vi "snr_test.vi"() -> ()   [LabVIEW 2017]
uses:
  <vilib>/measure/NI_MABase.lvlib
panel:
  in  "felharmonikus N":i32
  in  "noise (rms)":dbl format="%.2p"
  in  "zaj":bool
  out "kiolvasott frekvencia [Hz]":dbl
  in  "alh frekvencia [Hz]":dbl=10.0 format="%0.2p"
  in  "felh frekvencia [Hz]":dbl=10.0 format="%0.2p"
  out "Noise Integral":dbl
  out "Signal Integral":dbl
  out "SNR":dbl
  out "PSD":cluster{"f0":dbl, "df":dbl, "magnitude":dbl[]}[](graph)
  out "generált jel":waveform(dbl)(graph)
  in  "ablak szélesség [Hz]":dbl=20.0 format="%#_13g"
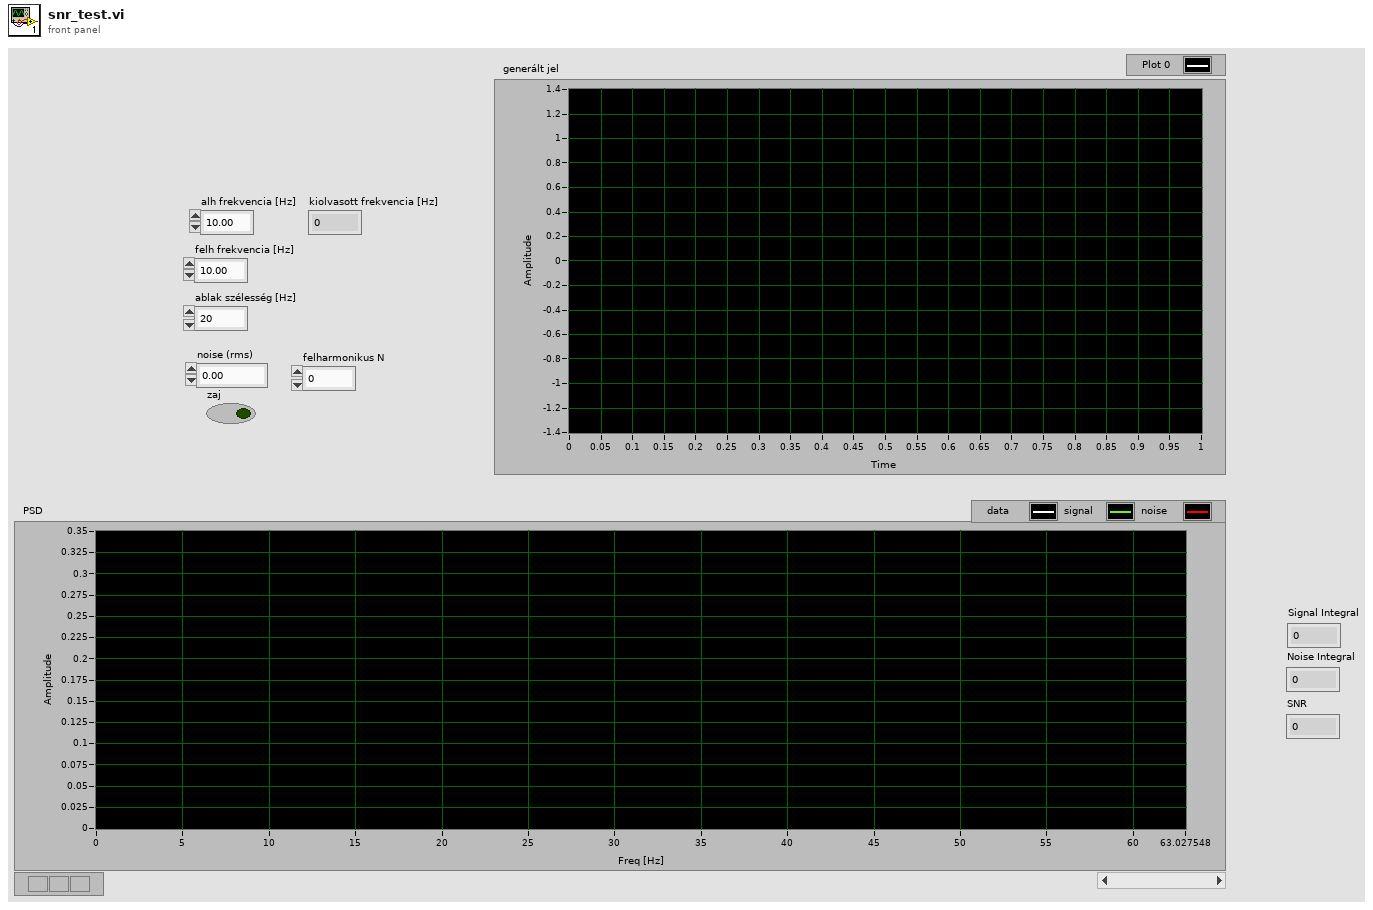
[diagram p1: front panel]
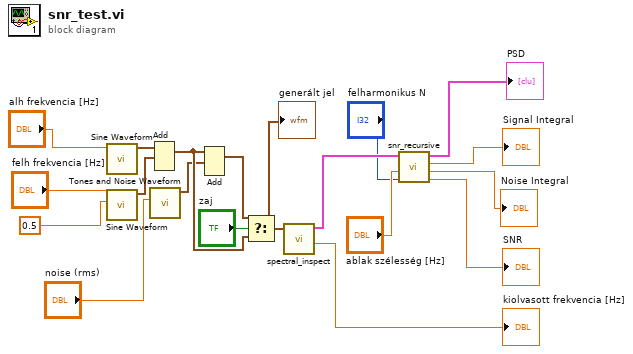
[diagram p0: block diagram]
diagram:
  n1 = call <vilib>:"Sine Waveform.vi"("frequency"="alh frekvencia [Hz]") -> ("signal out"=w17:waveform(dbl))  [unwired: 9 in, 1 out]
  n2 = call <vilib>:"Sine Waveform.vi"("amplitude"=0.5, "frequency"="felh frekvencia [Hz]") -> ("signal out"=w16:waveform(dbl))  [unwired: 8 in, 1 out]
  n3 = Add(1:w16, 2:w17) -> (0:w4:waveform(dbl))  [unwired: 1 in, 1 out]
  n4 = call <vilib>:"Tones and Noise Waveform.vi"("noise (rms)"="noise (rms)") -> ("signal out"=w3:waveform(dbl))  [unwired: 9 in, 1 out]
  n5 = Add(1:w3, 2:w4) -> (0:w5:waveform(dbl))  [unwired: 1 in, 1 out]
  n6 = Select(t=w5, s="zaj", f=w4) -> (s? t:f=w7:waveform(dbl))
  "generált jel" <- w7
  n7 = call "spectral_inspect.vi"("waveform"=w7) -> ("freq"=→"kiolvasott frekvencia [Hz]":dbl, "PSD"=w19:cluster{"f0":dbl, "df":dbl, "magnitude":dbl[]})  [unwired: 7 in, 2 out]
  n8 = call "snr_recursive.vi"("felharmonikus N"="felharmonikus N", "width [Hz]"="ablak szélesség [Hz]", "PSD"=w19) -> ("SNR"=→"SNR":dbl, "Noise Integral"=→"Noise Integral":dbl, "Signal Integral"=→"Signal Integral":dbl, "PSD"=→"PSD":cluster{"f0":dbl, "df":dbl, "magnitude":dbl[]}[])  [unwired: 5 in]
